vi "Process wallet.vi"(11 "Wallet contents":T1[](array[typedef])) -> (0 "Wallet total (£)":dbl, 1 "Indexes of next denom":i32[](array[numeric]), 2 "All my coins (values, £)":dbl[](array[numeric]), 3 "Wallet contents (dup)":T1[](array[typedef]), 5 "No. coins":i32)   [LabVIEW 2018]
uses:
  ctl/Coin data--cluster.ctl
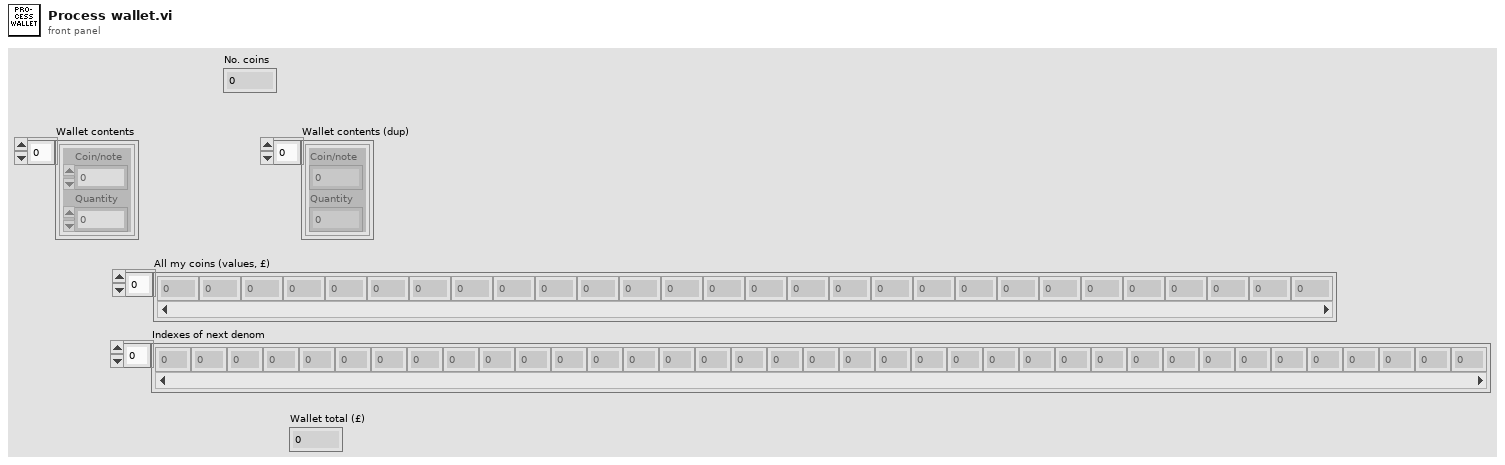
[diagram p1: front panel]
types:
  T1 = typedef "Coin data--cluster.ctl" = cluster{"Coin/note":i32, "Quantity":i32}
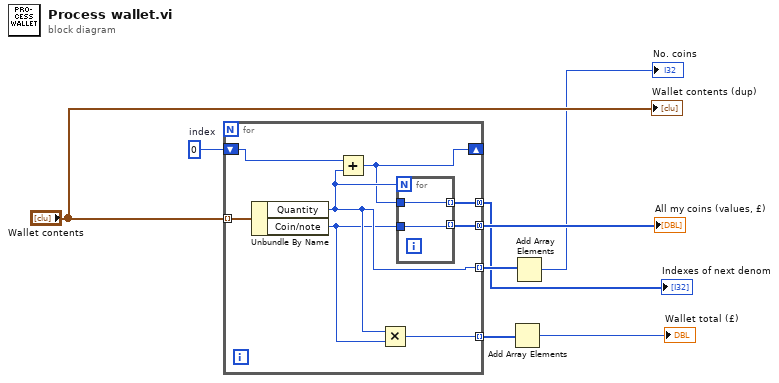
[diagram p0: block diagram]
diagram:
  w8 = 0  # index
  n1 = for {
    tunnel: "Wallet contents" -> [w16] mode=indexing
    shift-right: [w10] -> _
    shift-left: w8 -> [w15]
    tunnel: [w14] -> w3 mode=concatenating
    tunnel: [w13] -> w7 mode=indexing
    tunnel: [w11] -> w5 mode=indexing
    tunnel: [w9] -> w1 mode=concatenating
    n2 = Unbundle By Name(w16) -> ("Quantity"=w13:i32, "Coin/note"=w12:i32)
    n3 = Add(x=w15, y=w13) -> (x+y=w10:i32)
    n4 = Multiply(x=w13, y=w12) -> (x*y=w11:i32)
    n5 = for {
      N: w13 -> [_]
      tunnel: w12 -> [w18]
      tunnel: [w18] -> w14 mode=indexing
      tunnel: w10 -> [w17]
      tunnel: [w17] -> w9 mode=indexing
    }
  }
  "Indexes of next denom" <- w1
  "All my coins (values, £)" <- w3
  n6 = Add Array Elements(numeric array=w5) -> (sum=→"Wallet total (£)":i32)
  n7 = Add Array Elements(numeric array=w7) -> (sum=→"No. coins":i32)
  "Wallet contents (dup)" <- "Wallet contents"
